vi "Test MQTT-3.3.2-3.vi"(8 "error in (no error)":errorcluster) -> (0 "error out":errorcluster)   [LabVIEW 2013]
uses:
  source/Client/Client.lvclass/Client.ctl
  source/Control Packets/PUBLISH/PUBLISH.lvclass
  <vilib>/addons/_JKI Toolkits/Caraya/classes/Test/Test.lvclass
  source/Client/Client.lvclass
  <vilib>/addons/_JKI Toolkits/Caraya/classes/Assert/Assert.lvclass
  source/MQTT_Base/MQTT_Base.lvclass
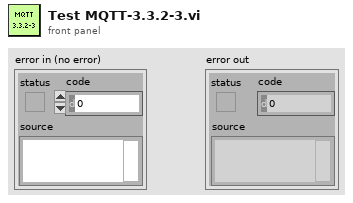
[diagram p1: front panel]
types:
  T1 = typedef "MQTT Server.lvlib/Client.lvclass/Public Events -- cluster.ctl" = cluster{"Connection Status":refnum<user-event>, "Connected":refnum<user-event>, "Application Message":refnum<user-event>}
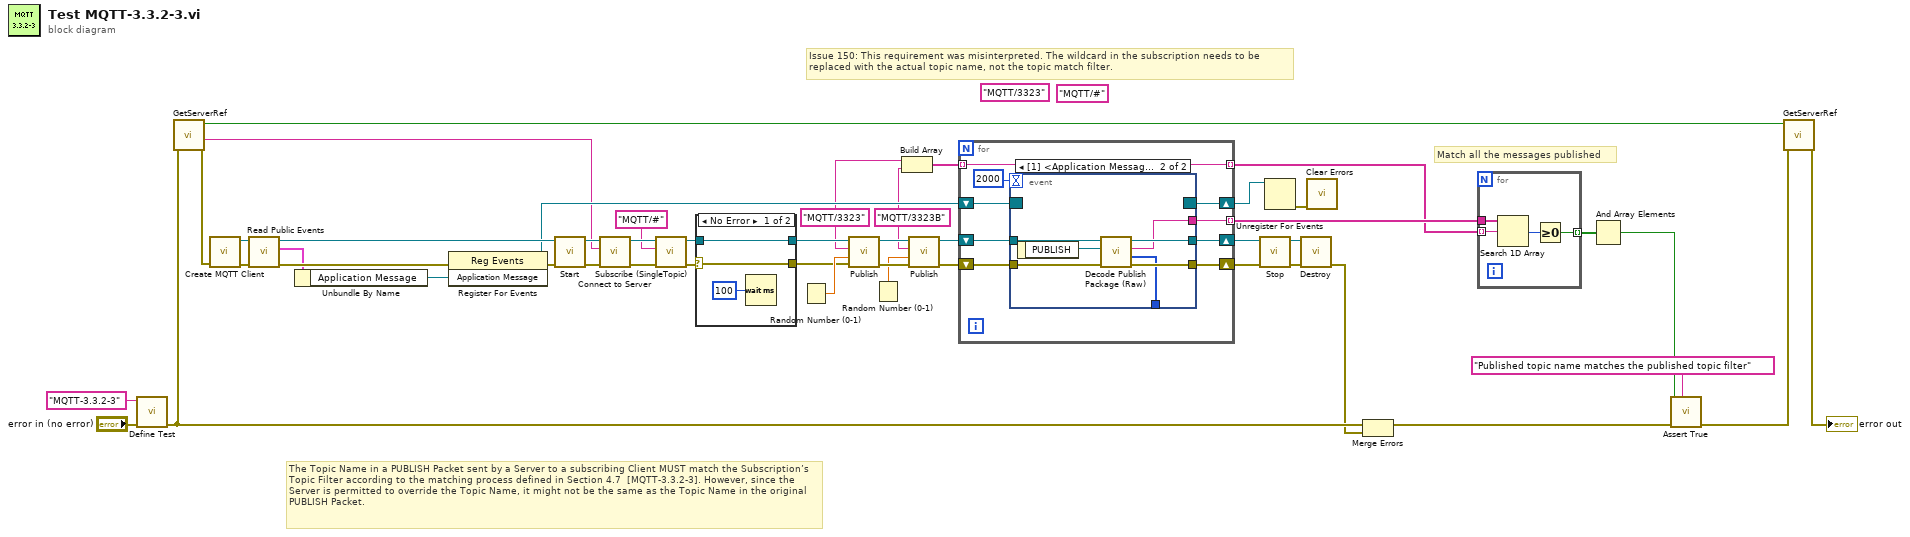
[diagram p0: block diagram]
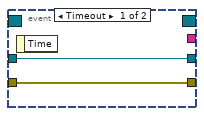
[diagram p2: hidden frame]
diagram:
  w3 = "MQTT/3323B" ("Topic Filter")
  (unwired) "MQTT/3323" ("Topic Filter")
  (unwired) "MQTT/#" ("Topic Filter")
  w4 = "MQTT/3323" ("Topic Filter")
  # "Match all the messages published"
  # "Issue 150: This requirement was misinterpreted. The wildcard in the subscription needs to be\nreplaced with the actual topic name, not the topic match filter."
  # "The Topic Name in a PUBLISH Packet sent by a Server to a subscribing Client MUST match the Subscription’s Topic Filter according to the matching process defined in Section 4.7  [MQTT-3.3.2-3]. However, since the Server is permitted to override the Topic Name, it might not be the same as the Topic Name in the original PUBLISH Packet."
  n1 = call <vilib>:"Define Test.vi"("error in (no error)"="error in (no error)", "Label (VI Title)"="MQTT-3.3.2-3") -> ("error out"=w40:errorcluster)  [unwired: 9 in]
  n2 = call "GetServerRef.vi"("error in"=w40) -> ("error out"=w44:errorcluster, "Server address"=w15:string, "Created"=w45:bool)  [unwired: 7 in, 1 out]
  n3 = call "Create MQTT Client.vi"("error in (no error)"=w44) -> ("error out"=w25:errorcluster, "Client out"=w27:refnum<class "Client.lvclass">)  [unwired: 9 in]
  n4 = call "Read Public Events.vi"("error in (no error)"=w25, "Client in"=w27) -> ("error out"=w24:errorcluster, "Client Public Events"=w23:T1, "Client out"=w26:refnum<class "Client.lvclass">)  [unwired: 7 in]
  n5 = Unbundle By Name(w23) -> ("Application Message"=w22:refnum<user-event>)
  n6 = register-events(error in=w24, w22) -> (reference out=w21:refnum<event-registration>, error out=w28:errorcluster)  [unwired: 1 in]
  n7 = call "Start.vi"("error in (no error)"=w28, "MQTT_Base in"=w26) -> ("error out"=w36:errorcluster, "MQTT_Base out"=w37:refnum<class "Client.lvclass">)  [unwired: 7 in, 1 out]
  n8 = call "Connect to Server.vi"("error in (no error)"=w36, "address (localhost)"=w15, "Client in"=w37) -> ("error out"=w34:errorcluster, "Client out"=w35:refnum<class "Client.lvclass">)  [unwired: 5 in, 2 out]
  n9 = call "Subscribe (SingleTopic).vi"("error in (no error)"=w34, "Topic Filter"="MQTT/#", "MQTT_Base in"=w35) -> ("error out"=w19:errorcluster, "MQTT_Base out"=w18:refnum<class "Client.lvclass">)  [unwired: 7 in]
  n10 = case shown="No Error" w19 {
    selector: w19 -> [w49 w51]
    tunnel: w18 -> [w50 w52]
    tunnel: [w50 w52] -> w17
    tunnel: [w49 w51] -> w16
    frame No Error {
      n11 = Wait (ms)(milliseconds to wait=u32 100) -> ()  [unwired: 1 out]
    }
    frame Error {
    }
  }
  n12 = Random Number (0-1)() -> (number: 0 to 1=w33:dbl)
  n13 = call "Publish.vi"("error in (no error)"=w16, "Payload"=w33, "Topic Name (empty: Payload name)"=w4, "Client in"=w17) -> ("error out"=w11:errorcluster, "Client out"=w13:refnum<class "Client.lvclass">)  [unwired: 5 in, 1 out]
  n14 = Random Number (0-1)() -> (number: 0 to 1=w9:dbl)
  n15 = Build Array(w4, w3) -> (w2:string[])
  n16 = call "Publish.vi"("error in (no error)"=w11, "Payload"=w9, "Topic Name (empty: Payload name)"=w3, "Client in"=w13) -> ("error out"=w10:errorcluster, "Client out"=w12:refnum<class "Client.lvclass">)  [unwired: 5 in, 1 out]
  n17 = for {
    shift-right: [w57] -> w20
    shift-left: w21 -> [w58]
    tunnel: [w54] -> w8 mode=indexing
    shift-right: [w59] -> w29
    shift-left: w12 -> [w56]
    shift-right: [w60] -> w30
    shift-left: w10 -> [w55]
    tunnel: w2 -> [w53] mode=indexing
    tunnel: [w53] -> w1 mode=indexing
    n18 = event shown="[1] <Application Message>: User Event" {
      selector: w58 -> [_ _]
      dyn-events: [_ _] -> w57
      timeout: 2000 -> [_ _]
      tunnel: w56 -> [w63 w70]
      tunnel: [w63 w68] -> w59
      tunnel: [w62 w67] -> w60
      tunnel: w55 -> [w62 w66]
      tunnel: [_ w65] -> _
      tunnel: [_ w64] -> w54
      event Timeout {
        n19 = event-data() -> ()  [unwired: 1 in, 1 out]
      }
      event User Event {
        n20 = event-data() -> ("PUBLISH"=w69:refnum<class "PUBLISH.lvclass">)  [unwired: 1 in]
        n21 = call "Decode Publish Package (Raw).vi"("error in (no error)"=w66, "PUBLISH in"=w69, "MQTT_Base in"=w70) -> ("error out"=w67:errorcluster, "Payload"=w65:u8[], "Topic"=w64:string, "MQTT_Base out"=w68:refnum<class "Client.lvclass">)  [unwired: 5 in]
      }
    }
  }
  n22 = call "Stop.vi"("error in (no error)"=w30, "MQTT_Base in"=w29) -> ("error out"=w31:errorcluster, "MQTT_Base out"=w32:refnum<class "Client.lvclass">)  [unwired: 7 in, 1 out]
  n23 = Unregister For Events(event registration refnum=w20) -> (error out=w14:errorcluster)  [unwired: 1 in]
  n24 = call "Destroy.vi"("error in (no error)"=w31, "MQTT_Base in"=w32) -> ("error out"=w38:errorcluster)  [unwired: 8 in, 1 out]
  n25 = call <vilib>:"Clear Errors.vi"("error in (no error)"=w14) -> ()  [unwired: 6 in, 1 out]
  n26 = Merge Errors(w40, w38) -> (w39:errorcluster)
  n27 = for {
    tunnel: w1 -> [w73] mode=indexing
    tunnel: w8 -> [w74]
    tunnel: [w71] -> w7 mode=indexing
    n28 = Search 1D Array(1D array=w74, element=w73) -> (index of element=w72:i32)  [unwired: 1 in]
    n29 = Greater Or Equal To 0?(x=w72) -> (x >= 0?=w71:bool)
  }
  n30 = And Array Elements(Boolean array=w7) -> (logical AND=w6:bool)
  n31 = call <vilib>:"Assert True.vi"("Label"="Published topic name matches the published topic filter", "error in (no error)"=w39, "True?"=w6) -> ("error out"=w43:errorcluster)  [unwired: 8 in]
  n32 = call "GetServerRef.vi"("error in"=w43, "Destroy (F)"=w45) -> ("error out"=→"error out":errorcluster)  [unwired: 6 in, 3 out]
